vi "B.vi"() -> ()   [LabVIEW 2010]
panel:
  out "received data":i32
  in  "stop":bool
  out "loop counter":i32
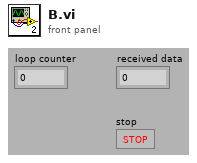
[diagram p1: front panel]
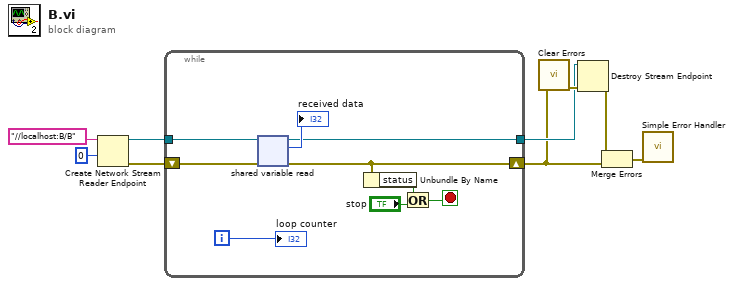
[diagram p0: block diagram]
diagram:
  n1 = Create Network Stream Reader Endpoint(9:0, 11:"//localhost:B/B" ("reader name")) -> (0:w9:errorcluster, 3:w8:refnum<k21>)  [unwired: 4 in]
  n2 = while {
    tunnel: w8 -> [w16]
    shift-right: [w14] -> w2
    shift-left: w9 -> [w17]
    tunnel: [w10] -> w3
    i -> [w18]
    stop <- w11 stop-if-true
    n3 = shared-variable-read(w16, w17) -> (w10:refnum<k21>, w14:errorcluster, →"received data":i32)  [unwired: 1 in, 1 out]
    n4 = Unbundle By Name(w14) -> ("status"=w13:bool)
    n5 = Or(x=w13, y="stop") -> (x .or. y?=w11:bool)
    "loop counter" <- w18
  }
  n6 = call <vilib>:"Clear Errors.vi"("error in (no error)"=w2) -> ("error out"=w5:errorcluster)  [unwired: 6 in]
  n7 = Destroy Stream Endpoint(8:w5, 11:w3) -> (0:w4:errorcluster)
  n8 = Merge Errors(w4, w2) -> (w1:errorcluster)
  n9 = call <vilib>:"Simple Error Handler.vi"("error in (no error)"=w1) -> ()  [unwired: 4 in, 5 out]
